vi "Fft-16.vi"() -> ()   [LabVIEW 2014]
uses:
  <vilib>/Platform/TimedLoop/XDataNode/timing_clust.ctl
  <vilib>/Platform/TimedLoop/XDataNode/nitl_modes.ctl
  <vilib>/Platform/TimedLoop/XDataNode/wakeup.ctl
  <vilib>/rvi/Analysis/measure/FFT/simModelSupport/niFPGA FFT Sim Properties.ctl
  <vilib>/rvi/Analysis/measure/FFT/simModelSupport/niFPGA FFT Sim Types.ctl
  <vilib>/rvi/Analysis/measure/FFT/simModelSupport/niFpgaFFTSimArithmeticProperties.ctl
  <vilib>/rvi/Analysis/measure/FFT/simModelSupport/niFpgaFFTSimDfxp.ctl
  <vilib>/fxp/LVFixedPointQuantizationPolicyTypeDef.ctl
  <vilib>/rvi/Emulation/niFpgaSctlEmulationGetInTimedLoop.vi
  <vilib>/rvi/Emulation/niFpgaEmulationReportErrorSimple.vi
  <vilib>/rvi/Emulation/niFpgaGetClockAttributes.vi
  <vilib>/rvi/Emulation/niFpgaCriticalErrorInLSC.vi
  <vilib>/rvi/interface/RandomDataEmulation/niFpgaRandomDataHandleErrors.vi
  <vilib>/rvi/Emulation/niFpgaEmulationIsFPGAContextNoSignature.vi
  <vilib>/rvi/errors/niFpgaSetErrorForExecOnDevCompSimple.vi
  <vilib>/rvi/eio/common/nirviEmuReportErrorAndStop.vi
  <vilib>/rvi/DataTransferAndStorage/Container/Common/niFpgaContainerGetUniqueNameForEmu.vi
  <vilib>/rvi/FIFO/Fifo_Resource/nirvififoEmulationSetSize.vi
  <vilib>/rvi/FIFO/Fifo_Resource/nirviFifoEmulationQueueMgr.vi
  <instcachedir>/0/nirviFifoEmulationQueueMgr_E5CAEC123FF24DC58D834DCA3CDAA9B5.lvgen/nirviFifoEmulationQueueMgr_E5CAEC123FF24DC58D834DCA3CDAA9B5_002.vi
  <vilib>/rvi/FIFO/Fifo_Resource/nirvififoEmulationDetermineInputValidOut.vi
  <vilib>/rvi/FIFO/Fifo_Resource/nirvififoEmulationCreateLock.vi
  <vilib>/rvi/Emulation/niFpgaProcessEmulError.vi
  <vilib>/rvi/FIFO/Fifo_Resource/nirvififoEmulationObtainLock.vi
  <vilib>/rvi/FIFO/Fifo_Resource/nirvififoEmulationReleaseLock.vi
  <vilib>/rvi/occurrence/nirviWaitOnOccurrenceBase.vi
  <vilib>/rvi/errors/nirviReportUnexpectedCaseInternalError.vi
  <vilib>/rvi/errors/nirviReportUnexpectedCaseInternalError (U32).vi
  <vilib>/Utility/error.llb/Clear Errors.vi
  <vilib>/rvi/Analysis/measure/FFT/simModelSupport/niFpgaFFTSimModelCore.vi
  <vilib>/Platform/TimedLoop/XDataNode/XDataNode.xnode
  <vilib>/rvi/DataTransferAndStorage/Container/XNode/niFpgaContainer.xnode
  <vilib>/rvi/interface/RandomDataEmulation/nirviRandomDataFpgaReadWriteTemplate.vi
  <vilib>/rvi/FIFO/Fifo_Resource/nirvififoEmulationWrite.vi
  <vilib>/rvi/FIFO/Fifo_Resource/nirvififoEmulationRead.vi
  <vilib>/rvi/Analysis/measure/FFT/XNode/niFpgaFFT.xnode
  <vilib>/Platform/TimedLoop/XDataNode/XDNodeRunTimeDep.lvlib
panel:
  out "Fft Size":u64
  out "output valid":bool
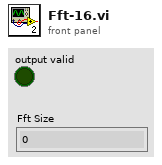
[diagram p1: front panel]
types:
  T1 = typedef "XDNodeRunTimeDep.lvlib/timing_clust.ctl" = cluster{"Expected End [f-1]":u64, "Actual End [f-1]":u64, "Finished Late? [f-1]":bool, "Expected End [i-1]":u64, "Actual End [i-1]":u64, "Finished Late? [i-1]":bool, "Expected Start [i]":u64, "Actual Start [i]":u64, "Expected Start [f]":u64, "Actual Start [f]":u64, "Source Name":string, "Structure Name":string, "Period":i64, "Deadline":i64, "Offset":i64, "Start":i64, "Priority":i32, "Timeout":i32, "Mode":T2, "Wakeup Reason":T3, "Error":errorcluster, "Source Type":string, "Secondary Source Type":string, "Global End Time":u64, "Global Start Time":u64, "Frame Duration":u64, "Iteration Duration":u64, "Assigned CPU":i32, "I/O Scan Engine Mode":u32}
  T2 = typedef "XDNodeRunTimeDep.lvlib/nitl_modes.ctl" = enum32{"No Change", "Process missed periods, maintain original phase", "Discard missed periods, maintain original phase", "Process missed periods, ignore original phase", "Discard missed periods, ignore original phase"}
  T3 = typedef "XDNodeRunTimeDep.lvlib/wakeup.ctl" = enum32{"Normal", "Aborted", "Asynchronous wakeup", "Timing source error", "Timed loop error", "Timeout"}
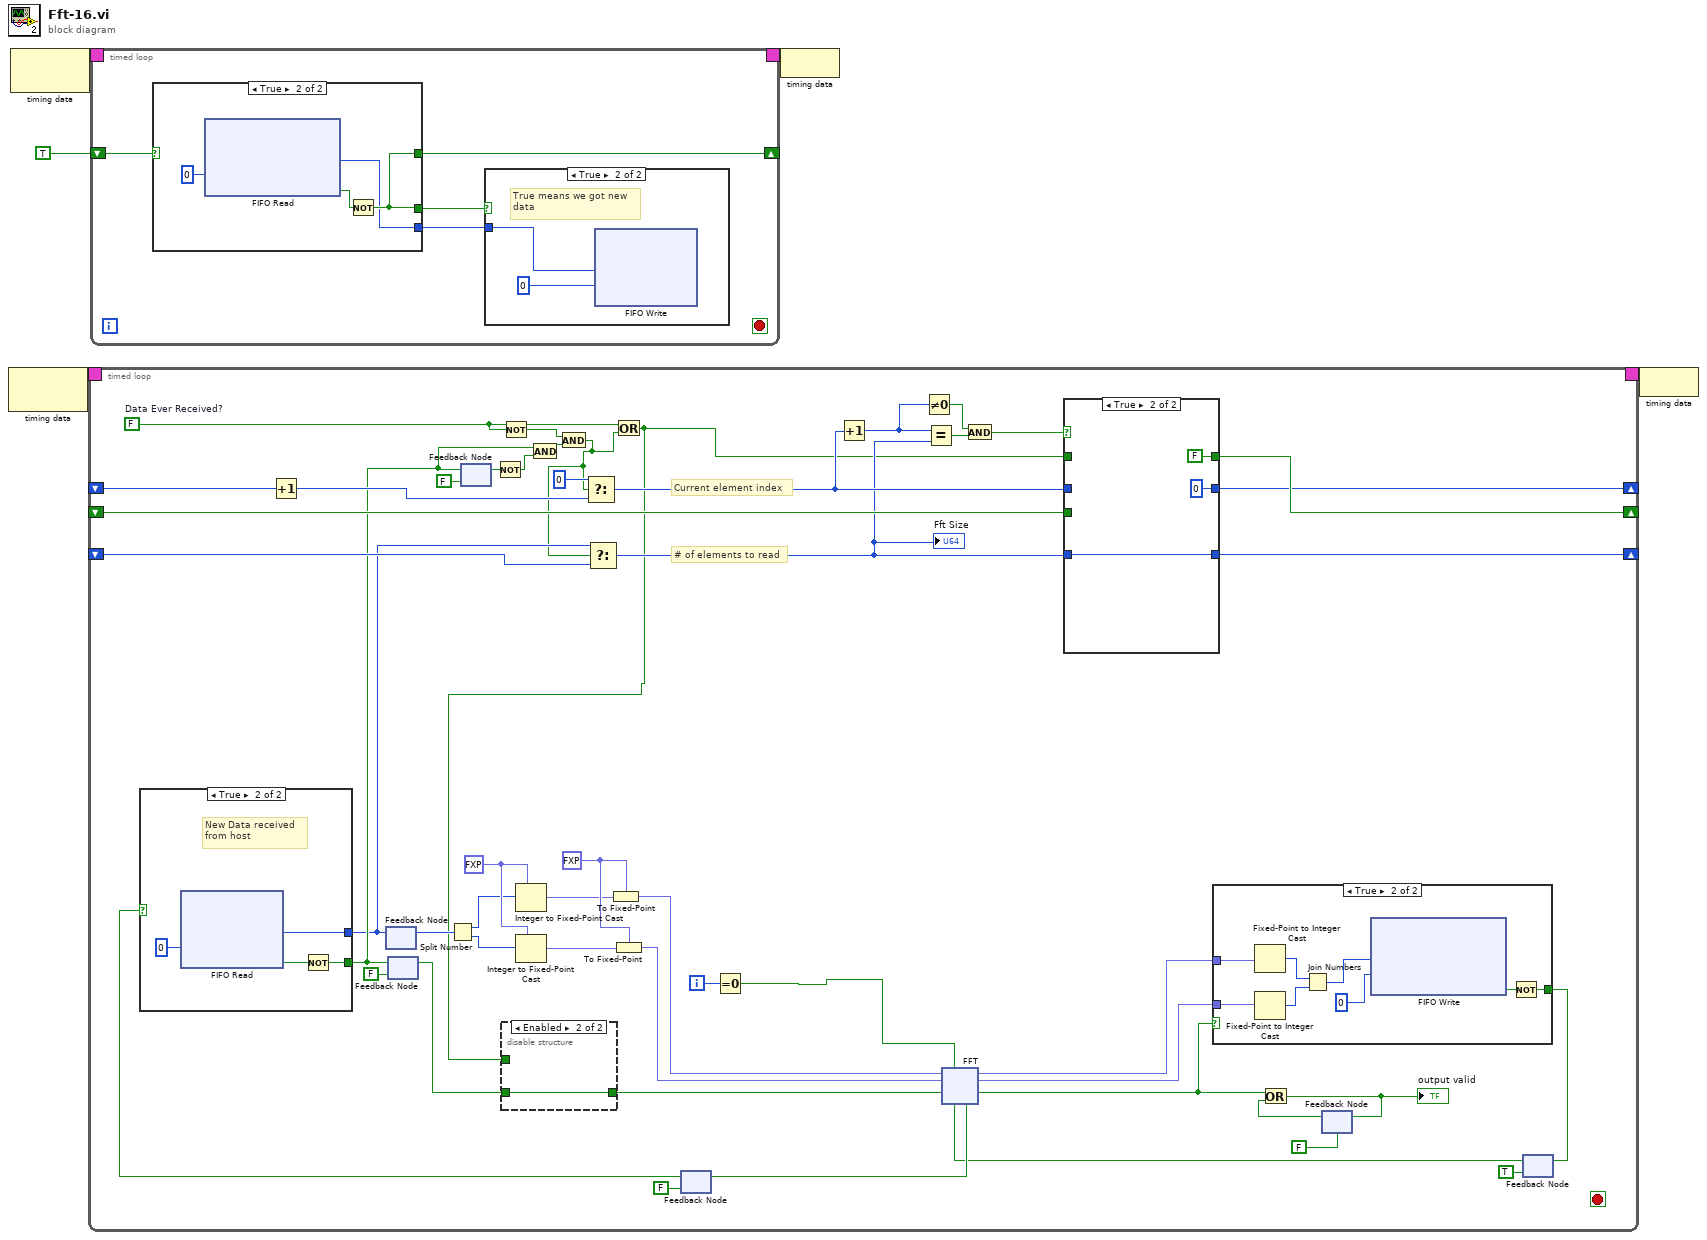
[diagram p0: block diagram]
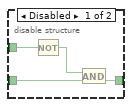
[diagram p2: hidden frame]
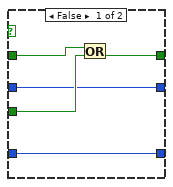
[diagram p3: hidden frame]
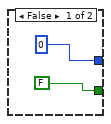
[diagram p4: hidden frame]
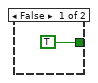
[diagram p5: hidden frame]
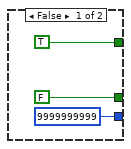
[diagram p7: hidden frame]
diagram:
  n1 = node-c288() -> (w2:T1)  [unwired: 1 in]
  n2 = node-c288() -> (w5:T1)  [unwired: 1 in]
  n3 = timed-loop {
    timing: w2 -> [_]
    timing-out: [_] -> w1
    shift-right: [w33] -> _
    shift-left: _ -> [w32]
    shift-right: [w26] -> _
    shift-left: _ -> [w25]
    shift-right: [w23] -> _
    shift-left: _ -> [w22]
    i -> [w45]
    stop <- _ stop-if-true
    w8 = FALSE  # Data Ever Received?
    w41 = fxp<+/-,24,7> 0.0 ("real data in")
    w44 = fxp<+/-,32,7> 0.0 ("real data in")
    # "Current element index"
    # "# of elements to read"
    n4 = Increment(x=w25) -> (x+1=w24:u32)
    n5 = feedback #1() -> (w17:u64)  [unwired: 1 in]
    n6 = feedback #2(FALSE ("Timed Out?")) -> (w29:bool)
    n7 = Split Number(x=w17) -> (hi(x)=w43:u32, lo(x)=w53:u32)
    n8 = feedback #3(FALSE ("Timed Out?")) -> (w30:bool)
    n9 = Not(x=w30) -> (.not. x?=w28:bool)
    n10 = Not(x=w8) -> (.not. x?=w7:bool)
    n11 = Integer to Fixed-Point Cast(fixed-point type=w44, integer=w43) -> (fixed-point=w38:fxp<+/-,32,7>)
    n12 = Integer to Fixed-Point Cast(fixed-point type=w44, integer=w53) -> (fixed-point=w39:fxp<+/-,32,7>)
    n13 = To Fixed-Point(fixed-point type=w41, number=w38) -> (fixed-point=w40:fxp<+/-,24,7>)
    n14 = To Fixed-Point(fixed-point type=w41, number=w39) -> (fixed-point=w42:fxp<+/-,24,7>)
    n15 = feedback #4(FALSE ("ready for data")) -> (w50:bool)
    n16 = case shown="True" w50 {
      tunnel: [FALSE ("Timed Out?") w100] -> w18
      tunnel: [u64 0 ("Element") w97] -> w16
      frame False {
      }
      frame True {
        # "New Data received \nfrom host"
        n17 = xnode ("FIFO Read")("Timeout"=0) -> ("Element"=w97:u64, "Timed Out?"=w98:bool)  [unwired: 1 in, 1 out]
        n18 = Not(x=w98) -> (.not. x?=w100:bool)
      }
    }
    n19 = feedback-in #1(w16) -> ()
    n20 = feedback-in #2(w18) -> ()
    n21 = feedback-in #3(w18) -> ()
    n22 = And(x=w18, y=w28) -> (x .and. y?=w10:bool)
    n23 = And(x=w7, y=w10) -> (x .and. y?=w9:bool)
    n24 = Select(t=u32 0, s=w9, f=w24) -> (s? t:f=w21:u32)
    n25 = Select(t=w16, s=w9, f=w22) -> (s? t:f=w13:u64)
    "Fft Size" <- w13
    n26 = Or(x=w8, y=w9) -> (x .or. y?=w11:bool)
    n27 = disable-structure shown="Enabled" {
      disable-tunnel: w29 -> [w59 w60]
      disable-tunnel: [w58 w60] -> w15
      disable-tunnel: w11 -> [w56 _]
      frame Disabled {
        n28 = Not(x=w56) -> (.not. x?=w57:bool)
        n29 = And(x=w57, y=w59) -> (x .and. y?=w58:bool)
      }
      frame Enabled {
      }
    }
    n30 = Equal To 0?(x=w45) -> (x = 0?=w6:bool)
    n31 = Increment(x=w21) -> (x+1=w12:u32)
    n32 = Not Equal To 0?(x=w12) -> (x != 0?=w19:bool)
    n33 = Equal?(x=w12, y=w13) -> (x = y?=w20:bool)
    n34 = And(x=w19, y=w20) -> (x .and. y?=w14:bool)
    n35 = case shown="True" w14 {
      tunnel: w11 -> [w89 _]
      tunnel: [w90 FALSE ("Data Ever Received?")] -> w33
      tunnel: w32 -> [w91 _]
      tunnel: w21 -> [w88 _]
      tunnel: [w88 u32 0] -> w26
      tunnel: w13 -> [w87 w92]
      tunnel: [w87 w92] -> w23
      frame False {
        n36 = Or(x=w89, y=w91) -> (x .or. y?=w90:bool)
      }
      frame True {
      }
    }
    n37 = feedback #5(FALSE) -> (w47:bool)
    n38 = feedback #6(TRUE ("Timed Out?")) -> (w51:bool)
    n39 = xnode "FFT"("real data in"=w40, "reset"=w6, "imaginary data in"=w42, "input valid"=w15, "ready for output"=w51) -> ("ready for input"=w54:bool, "real data out"=w36:fxp<+/-,32,12>, "imaginary data out"=w35:fxp<+/-,32,12>, "output valid"=w37:bool)  [unwired: 1 out]
    n40 = feedback-in #4(w54) -> ()
    n41 = case shown="True" w37 {
      tunnel: w36 -> [_ w102]
      tunnel: w35 -> [_ w107]
      tunnel: [TRUE ("Timed Out?") w103] -> w52
      frame False {
      }
      frame True {
        n42 = Fixed-Point to Integer Cast(1:w102) -> (0:w109:i32)
        n43 = Fixed-Point to Integer Cast(1:w107) -> (0:w108:i32)
        n44 = Join Numbers(hi=w109, lo=w108) -> ((hi.lo)=w106:u64)
        n45 = xnode ("FIFO Write")("Element"=w106, "Timeout"=0) -> ("Timed Out?"=w104:bool)  [unwired: 1 in, 1 out]
        n46 = Not(x=w104) -> (.not. x?=w103:bool)
      }
    }
    n47 = Or(x=w37, y=w47) -> (x .or. y?=w46:bool)
    "output valid" <- w46
    n48 = feedback-in #5(w46) -> ()
    n49 = feedback-in #6(w52) -> ()
  }
  n50 = timed-loop {
    timing: w5 -> [_]
    timing-out: [_] -> w4
    shift-right: [w113] -> _
    shift-left: TRUE -> [w115]
    stop <- _ stop-if-true
    n51 = case shown="True" w115 {
      tunnel: [TRUE w124] -> w113
      tunnel: [u64 9999999999 ("Element") w121] -> w114
      tunnel: [FALSE w124] -> w112
      frame False {
      }
      frame True {
        n52 = xnode ("FIFO Read")("Timeout"=0) -> ("Element"=w121:u64, "Timed Out?"=w122:bool)  [unwired: 1 in, 1 out]
        n53 = Not(x=w122) -> (.not. x?=w124:bool)
      }
    }
    n54 = case shown="True" w112 {
      tunnel: w114 -> [_ w116]
      frame False {
      }
      frame True {
        # "True means we got new\ndata"
        n55 = xnode ("FIFO Write")("Element"=w116, "Timeout"=0) -> ()  [unwired: 1 in, 2 out]
      }
    }
  }
  n56 = node-c288(w4) -> ()
  n57 = node-c288(w1) -> ()
